vi "subvi1.vi"(2 "reference":refnum<vi>, 3 "Array in":refnum<vi>) -> ()   [LabVIEW 2018]
uses:
  <vilib>/Utility/file.llb/Write Delimited Spreadsheet (DBL).vi
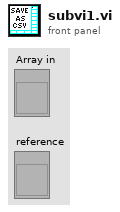
[diagram p1: front panel]
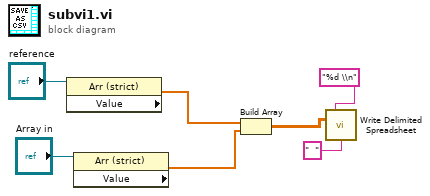
[diagram p0: block diagram]
diagram:
  n1 = property class="Arr (strict)"(reference="reference") -> ("Value"=w5:dbl[])  [unwired: 1 in, 2 out]
  n2 = property class="Arr (strict)"(reference="Array in") -> ("Value"=w6:dbl[])  [unwired: 1 in, 2 out]
  n3 = Build Array(w5, w6) -> (w3:dbl[][])
  n4 = call-poly <vilib>:"Write Delimited Spreadsheet.vi"("format (%.3f)"="%d \\n", "2D data"=w3, "delimiter (\\t)"="  " ("delimiter (\\t)")) -> ()  [unwired: 11 in, 2 out]
